vi "Initialize.vi"(8 "error in (no error)":errorcluster, 9 "ID Query":bool, 10 "Reset":bool, 11 "Tektronix DMM4020 in":refnum<class "Tektronix DMM4020.lvclass">) -> (0 "error out":errorcluster, 2 "VISA resource name":refnum<visa-resource-name>, 3 "Tektronix DMM4020 out":refnum<class "Tektronix DMM4020.lvclass">)   [LabVIEW 2014, in "Tektronix DMM4020.lvclass"]
uses:
  Tektronix DMM4020.lvclass
  <instrlib>/Tektronix DMM4020/Tektronix DMM4020.lvlib
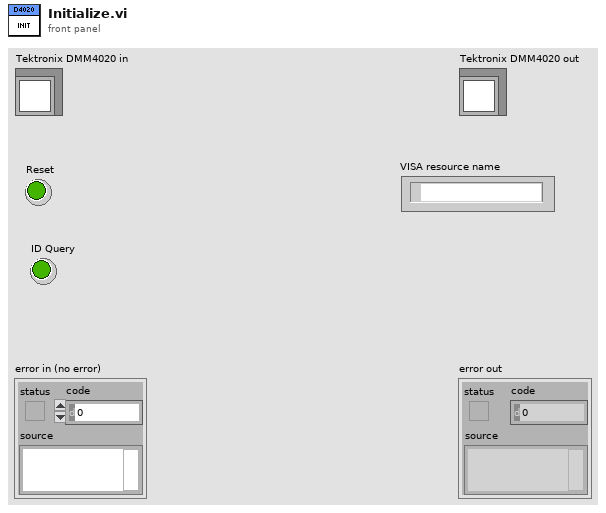
[diagram p1: front panel]
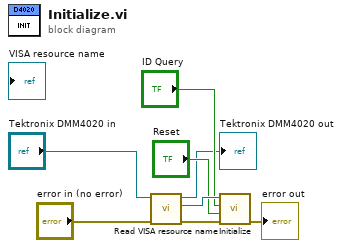
[diagram p0: block diagram]
diagram:
  n1 = call-dynamic "Read VISA resource name.vi"("error in (no error)"="error in (no error)", "Generic Instrument in"="Tektronix DMM4020 in") -> ("error out"=w3:errorcluster, "VISA resource name"=w7:refnum<visa-resource-name>, "Generic Instrument out"=→"Tektronix DMM4020 out":refnum<class "Tektronix DMM4020.lvclass">)  [unwired: 7 in]
  n2 = call <instrlib>:"Initialize.vi"("error in (no error)"=w3, "Reset (True)"="Reset", "ID Query (True)"="ID Query", "VISA resource name"=w7) -> ("error out"=→"error out":errorcluster)  [unwired: 5 in, 2 out]
